vi "Start.vi"(8 "error in (no error)":errorcluster, 11 "AODAcq in":refnum<class "AODAcq.lvclass">) -> (0 "error out":errorcluster, 3 "AODAcq out":refnum<class "AODAcq.lvclass">)   [LabVIEW 2011, in "AODAcq.lvclass"]
uses:
  AODAcq.lvclass
  AODAcq.lvclass/AODAcq.ctl
  <instrlib>/niHWS/nihws.llb/niHWS Set Wfm String Attribute ID.ctl
  <instrlib>/niHWS/nihws.llb/niHWS Set Wfm DBL Attribute.vi
  <vilib>/Utility/error.llb/Error Cluster From Error Code.vi
  <vilib>/rvi/errors/niLvFpgaAdjustHostInterfaceError.vi
  Program Files/National Instruments/LabVIEW 2011/Targets/NI/FPGA/StockFPGA_IntfPrivate/ScriptTemplates/StockFPGA_PlugInRead32.vi
  <vilib>/rvi/interface/nirviMethod/nirviMethod.xnode
  FPGA_Control/AODRef.ctl
  FPGA Bitfiles/Acquisition_FPGATarget_AODControl(FPGA)_C1C38267.lvbitx
  FPGA_Control/AOD Control (FPGA).vi
  <vilib>/rvi/interface/nirviReadWriteControl/nirviReadWriteControl.xnode
  <vilib>/rvi/errors/niLvFpgaMergeErrorWithErrorCode.vi
  <vilib>/FPGAPlugInAG/PXIe-7965R/niLvFpga_ReadFifo_PXIe-7965R.vi
  NiFpgaLv.dll
  <vilib>/FPGAPlugInAG/PXIe-7965R/niLvFpga_Read32_PXIe-7965R.vi
  <vilib>/rvi/interface/nirviReadWriteControl/niFpgaRWControlAccessTimeoutTemplate.vi
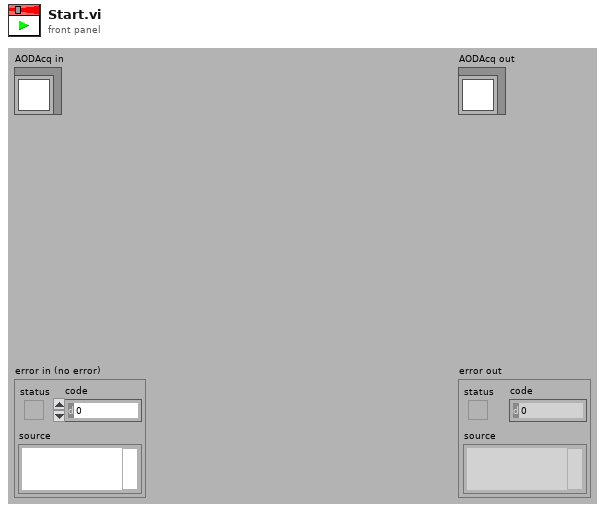
[diagram p1: front panel]
types:
  T1 = typedef "AODRef.ctl" = refnum<k20>
  T2 = typedef "niHWS Set Wfm String Attribute ID.ctl" = u32
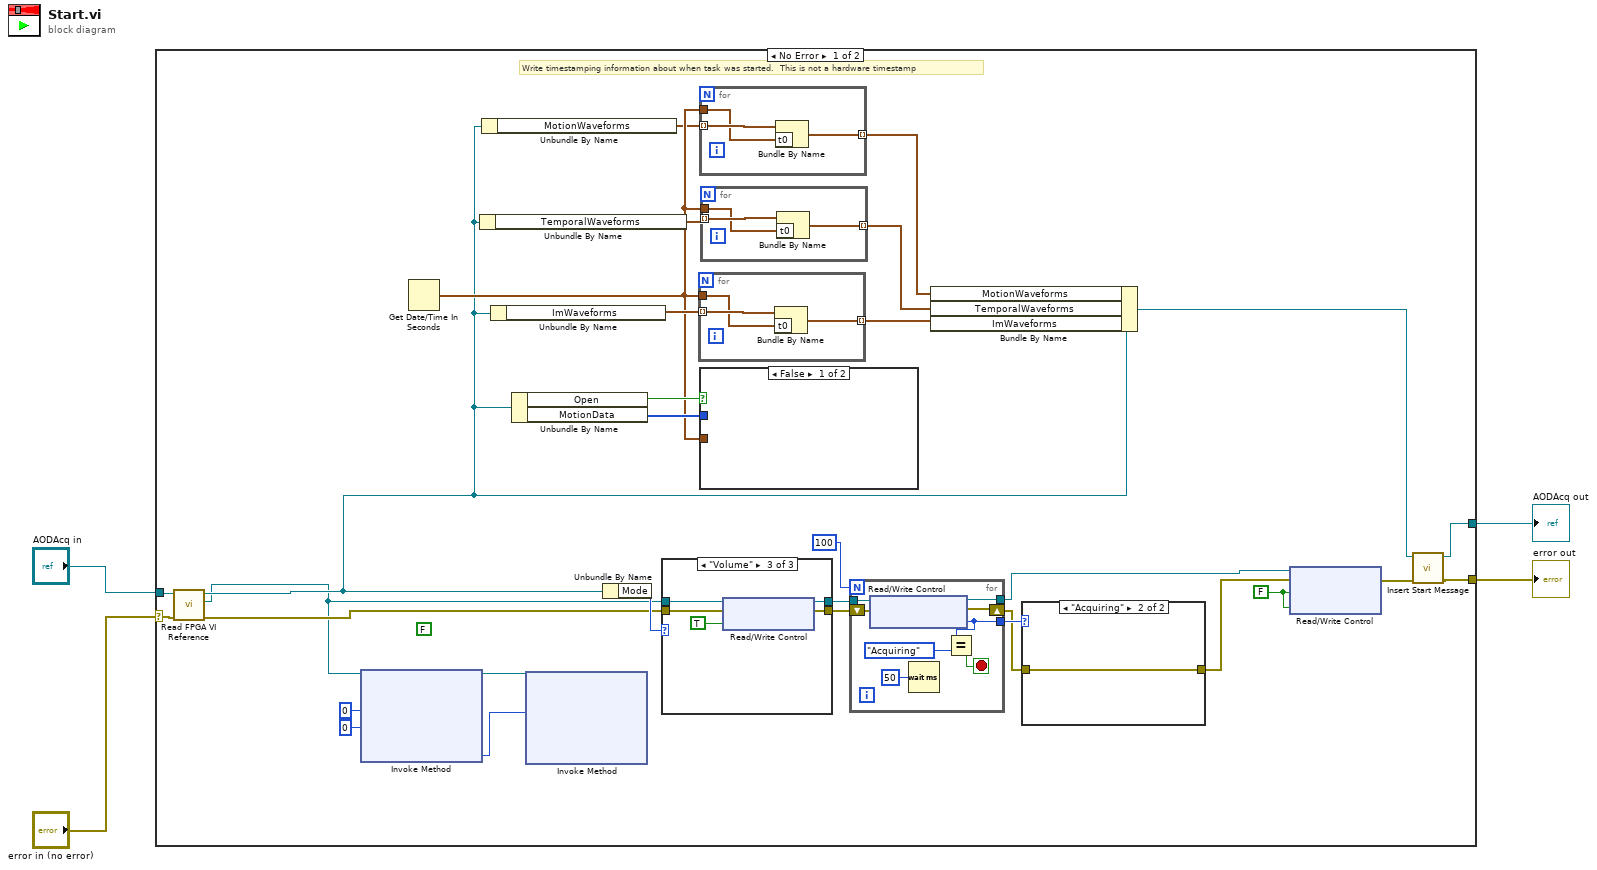
[diagram p0: block diagram]
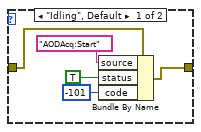
[diagram p2: hidden frame]
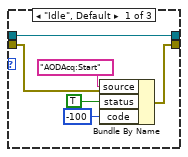
[diagram p3: hidden frame]
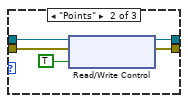
[diagram p4: hidden frame]
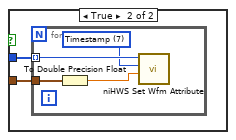
[diagram p5: hidden frame]
diagram:
  n1 = case shown="No Error" "error in (no error)" {
    selector: "error in (no error)" -> [w34 w82]
    tunnel: [w8 w82] -> w3
    tunnel: [w5 w81] -> w1
    tunnel: "AODAcq in" -> [w35 w81]
    frame No Error {
      w15 = FALSE ("ExtAcqTrig")
      (unwired) FALSE ("ExtAcqTrig")
      # "Write timestamping information about when task was started.  This is not a hardware timestamp"
      n2 = call-dynamic "Read FPGA VI Reference.vi"("error in (no error)"=w34, "AODAcq in"=w35) -> ("error out"=w14:errorcluster, "FPGA VI Reference"=w13:T1, "AODAcq out"=w16:refnum<class "AODAcq.lvclass">)  [unwired: 7 in]
      n3 = xnode "Invoke Method"("FPGA VI Reference In"=w13, "Number of Elements"=u32 0, "Timeout (ms)"=0) -> ("FPGA VI Reference Out"=w23:T1, "Elements Remaining"=w22:u32)  [unwired: 1 in, 2 out]
      n4 = Get Date/Time In Seconds() -> (seconds since 1Jan1904=w21:timestamp)
      n5 = Unbundle By Name(w16) -> ("TemporalWaveforms"=w20:waveform(i32)[])
      n6 = Unbundle By Name(w16) -> ("MotionWaveforms"=w19:waveform(i32)[])
      n7 = Unbundle By Name(w16) -> ("ImWaveforms"=w33:waveform(i32)[])
      n8 = Unbundle By Name(w16) -> ("Open"=w31:bool, "MotionData"=w30:u32[])
      n9 = xnode "Invoke Method"("FPGA VI Reference In"=w23, "Number of Elements"=w22) -> ()  [unwired: 2 in, 4 out]
      n10 = Unbundle By Name(w16) -> ("Mode"=w29:enum16{"Idle", "Points", "Volume"})
      n11 = case shown="\"Volume\"" w29 {
        tunnel: w13 -> [w61 w66 w70]
        tunnel: [w61 w65 w69] -> w26
        tunnel: [w57 w63 w68] -> w27
        tunnel: w14 -> [w56 w62 w67]
        frame "Idle", Default {
          n12 = Bundle By Name(cluster=w56, "source"="AODAcq:Start", "status"=TRUE, "code"=-100) -> (w57:errorcluster)
        }
        frame "Points" {
          n13 = xnode "Read/Write Control"("FPGA VI Reference In"=w66, "error in"=w62, "Control.Points"=TRUE) -> ("FPGA VI Reference Out"=w65:T1, "error out"=w63:errorcluster)
        }
        frame "Volume" {
          n14 = xnode "Read/Write Control"("FPGA VI Reference In"=w70, "error in"=w67, "Control.Volume"=TRUE ("Control.Points")) -> ("FPGA VI Reference Out"=w69:T1, "error out"=w68:errorcluster)
        }
      }
      n15 = for {
        tunnel: w33 -> [w80] mode=indexing
        tunnel: w21 -> [w79]
        tunnel: [w78] -> w32 mode=indexing
        n16 = Bundle By Name(cluster=w80, "t0"=w79) -> (w78:waveform(i32))
      }
      n17 = for {
        tunnel: w19 -> [w38] mode=indexing
        tunnel: w21 -> [w37]
        tunnel: [w36] -> w17 mode=indexing
        n18 = Bundle By Name(cluster=w38, "t0"=w37) -> (w36:waveform(i32))
      }
      n19 = case shown="False" w31 {
        tunnel: w30 -> [_ w73]
        tunnel: w21 -> [_ w72]
        frame False {
        }
        frame True {
          n20 = for {
            tunnel: w73 -> [w77] mode=indexing
            tunnel: w72 -> [w75]
            w76 = T2 7 items=["Note"=0, "X Axis Label"=1, "Y Axis Label"=2, "X Axis Units"=3, "Y Axis Units"=4, "Valid Signals"=6, "Timestamp"=7] ("attribute ID")
            n21 = To Double Precision Float(number=w75) -> (double precision float=w74:dbl)
            n22 = call-poly <instrlib>:"niHWS Set Wfm Attribute.vi"("attribute value"=w74, "attribute ID"=w76, "waveform reference in"=w77) -> ()  [unwired: 7 in, 2 out]
          }
        }
      }
      n23 = for {
        tunnel: w20 -> [w41] mode=indexing
        tunnel: w21 -> [w40]
        tunnel: [w39] -> w18 mode=indexing
        n24 = Bundle By Name(cluster=w41, "t0"=w40) -> (w39:waveform(i32))
      }
      n25 = for {
        N: 100 -> [_]
        tunnel: w26 -> [w55]
        tunnel: [w54] -> w10
        shift-right: [w48] -> w11
        shift-left: w27 -> [w52]
        tunnel: [w49] -> w12
        stop <- w50 stop-if-true
        n26 = xnode "Read/Write Control"("FPGA VI Reference In"=w55, "error in"=w52) -> ("FPGA VI Reference Out"=w54:T1, "error out"=w48:errorcluster, "Status.AcqState"=w49:enum16{"Idling", "Acquiring"})
        n27 = Wait (ms)(milliseconds to wait=u32 50) -> ()  [unwired: 1 out]
        n28 = Equal?(x=w49, y=enum16{"Idling", "Acquiring"}."Acquiring") -> (x = y?=w50:bool)
      }
      n29 = Bundle By Name(cluster=w16, "MotionWaveforms"=w17, "TemporalWaveforms"=w18, "ImWaveforms"=w32) -> (w6:refnum<class "AODAcq.lvclass">)
      n30 = case shown="\"Acquiring\"" w12 {
        tunnel: [w43 w47] -> w9
        tunnel: w11 -> [w42 w47]
        frame "Idling", Default {
          n31 = Bundle By Name(cluster=w42, "source"="AODAcq:Start", "status"=TRUE, "code"=-101) -> (w43:errorcluster)
        }
        frame "Acquiring" {
        }
      }
      n32 = xnode "Read/Write Control"("FPGA VI Reference In"=w10, "error in"=w9, "Control.Points"=w15, "Control.Volume"=w15) -> ("error out"=w7:errorcluster)  [unwired: 1 out]
      n33 = call-dynamic "Insert Start Message.vi"("error in (no error)"=w7, "AODAcq in"=w6) -> ("error out"=w8:errorcluster, "AODAcq out"=w5:refnum<class "AODAcq.lvclass">)  [unwired: 8 in]
    }
    frame Error {
    }
  }
  "error out" <- w3
  "AODAcq out" <- w1
